vi "Get.vi"(7 "Process Name":string, 8 "error in (no error)":errorcluster) -> (0 "error out":errorcluster, 3 "queue out":T1)   [LabVIEW 2016, in "System.lvlib"]
uses:
  System.lvlib
  Controls/Control_Queue Reference.ctl
  Controls/Control_Message Data.ctl
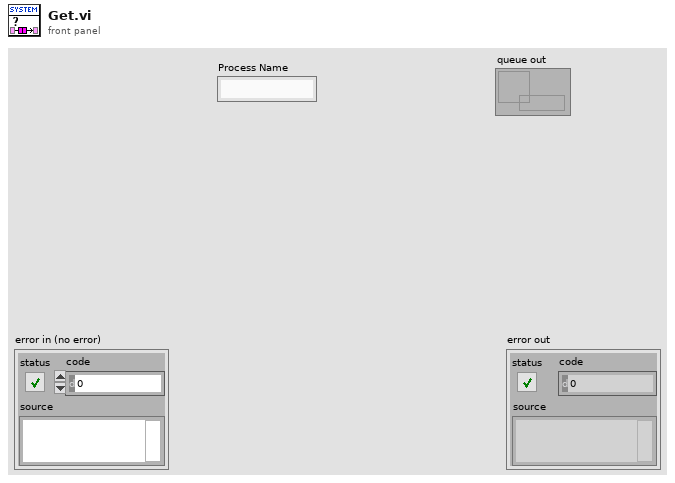
[diagram p1: front panel]
types:
  T1 = typedef "System.lvlib/Control_Queue Reference.ctl" = refnum<queue>
  T2 = typedef "System.lvlib/Control_Variant Data Reference.ctl" = refnum<data-value>
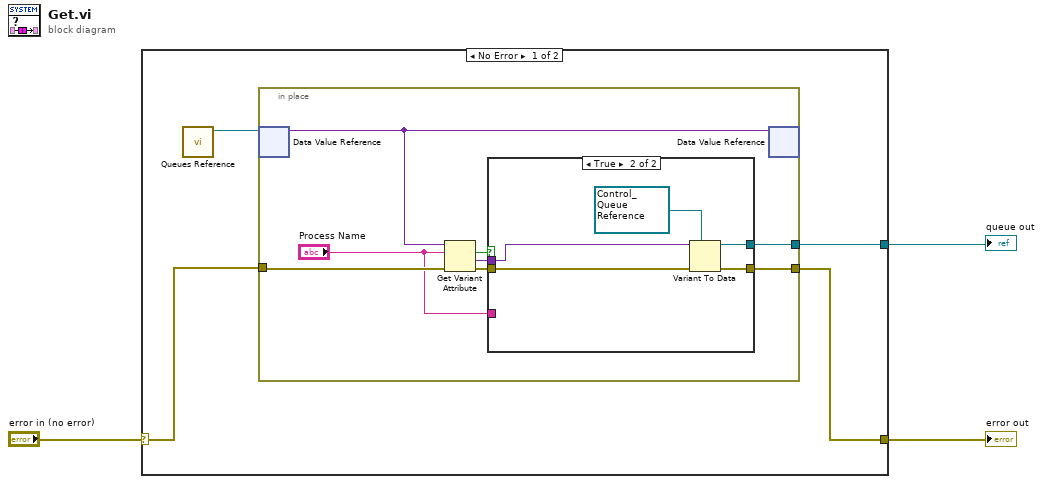
[diagram p0: block diagram]
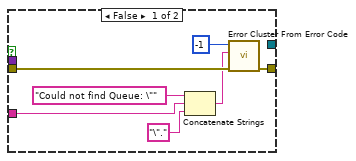
[diagram p2: hidden frame]
diagram:
  n1 = case shown="No Error" "error in (no error)" {
    selector: "error in (no error)" -> [w6 w28]
    tunnel: [w5 w28] -> w2
    tunnel: [w4 _] -> w1
    frame No Error {
      n2 = call "Queues Reference.vi"() -> ("Queues Reference"=w7:T2)  [unwired: 10 in, 1 out]
      n3 = in-place {
        in-place-border: w6 -> [w15]
        in-place-border: [w11] -> w4
        in-place-border: [w10] -> w5
        n4 = in-place-dvr #1(w7) -> (w8:variant)  [unwired: 1 out]
        n5 = Get Variant Attribute(Variant=w8, name="Process Name", error in=w15) -> (found=w14:bool, value=w13:variant, error out=w12:errorcluster)  [unwired: 1 in, 1 out]
        n6 = case shown="True" w14 {
          tunnel: w13 -> [_ w26]
          tunnel: w12 -> [w22 w27]
          tunnel: [_ w25] -> w11
          tunnel: [w21 w24] -> w10
          tunnel: "Process Name" -> [w18 _]
          frame False {
            n7 = Concatenate Strings("Could not find Queue: \"", w18, "\".") -> (w16:string)
            n8 = call <vilib>:"Error Cluster From Error Code.vi"("error in (no error)"=w22, "error message (\"\")"=w16, "error code (0)"=-1) -> ("error out"=w21:errorcluster)  [unwired: 6 in]
          }
          frame True {
            n9 = Variant To Data(error in=w27, type=T1 refnum ("queue"), Variant=w26) -> (data=w25:T1, error out=w24:errorcluster)
          }
        }
        n10 = in-place-dvr #1(w8) -> ()  [unwired: 2 out]
      }
    }
    frame Error {
    }
  }
  "error out" <- w2
  "queue out" <- w1
